vi "Madgwick Test.vi"() -> ()   [LabVIEW 2021]
uses:
  Lab 5/Lab 5 Code/Heading_TDef.ctl
  <vilib>/Platform/TimedLoop/XDataNode/timing_clust.ctl
  <vilib>/Platform/TimedLoop/XDataNode/nitl_modes.ctl
  <vilib>/Platform/TimedLoop/XDataNode/wakeup.ctl
  <vilib>/platform/TimedLoop/XDataNode/XDataNode.xnode
  <vilib>/Platform/TimedLoop/XDataNode/XDNodeRunTimeDep.lvlib
  Labview MadgwickAhrs/MadgwickOrientationFilter.lvlib
panel:
  out "Count":i32
  out "OrthogonalMatrix":dbl[][](array[numeric])
  out "Madgwick Conversion":cluster{"X":sgl, "Y":sgl, "Z":sgl}(graph)
  out "# elements in queue":i32
  out "Output Producer":dbl[][](array[numeric])
  out "Input Consumer":dbl[][](array[numeric])
  out "Quaternion":dbl[](array[numeric])
  out "Waveform Chart":waveform(dbl)[](graph)
  out "Gyro Output Offset Array (int)":i16[](array[numeric])
  in  "error in (no error)":errorcluster
  out "Mag Flux (uT)":T1(graph)
  out "Heading Output (Str)":T2
  out "Heading":dbl
  in  "Reset Gyro":bool
  out "Acceleration (g)":T3(graph)
  out "Velocity":T1(graph)
  out "Gyro Integration":T3(graph)
  out "Acceleration (ms^2)":dbl[](array[numeric])
  out "Velocity Cluster Out":cluster{i16, i16, i16}
  out "Rotation Cluster Out":T4
  out "error out":errorcluster
  in  "stop":bool
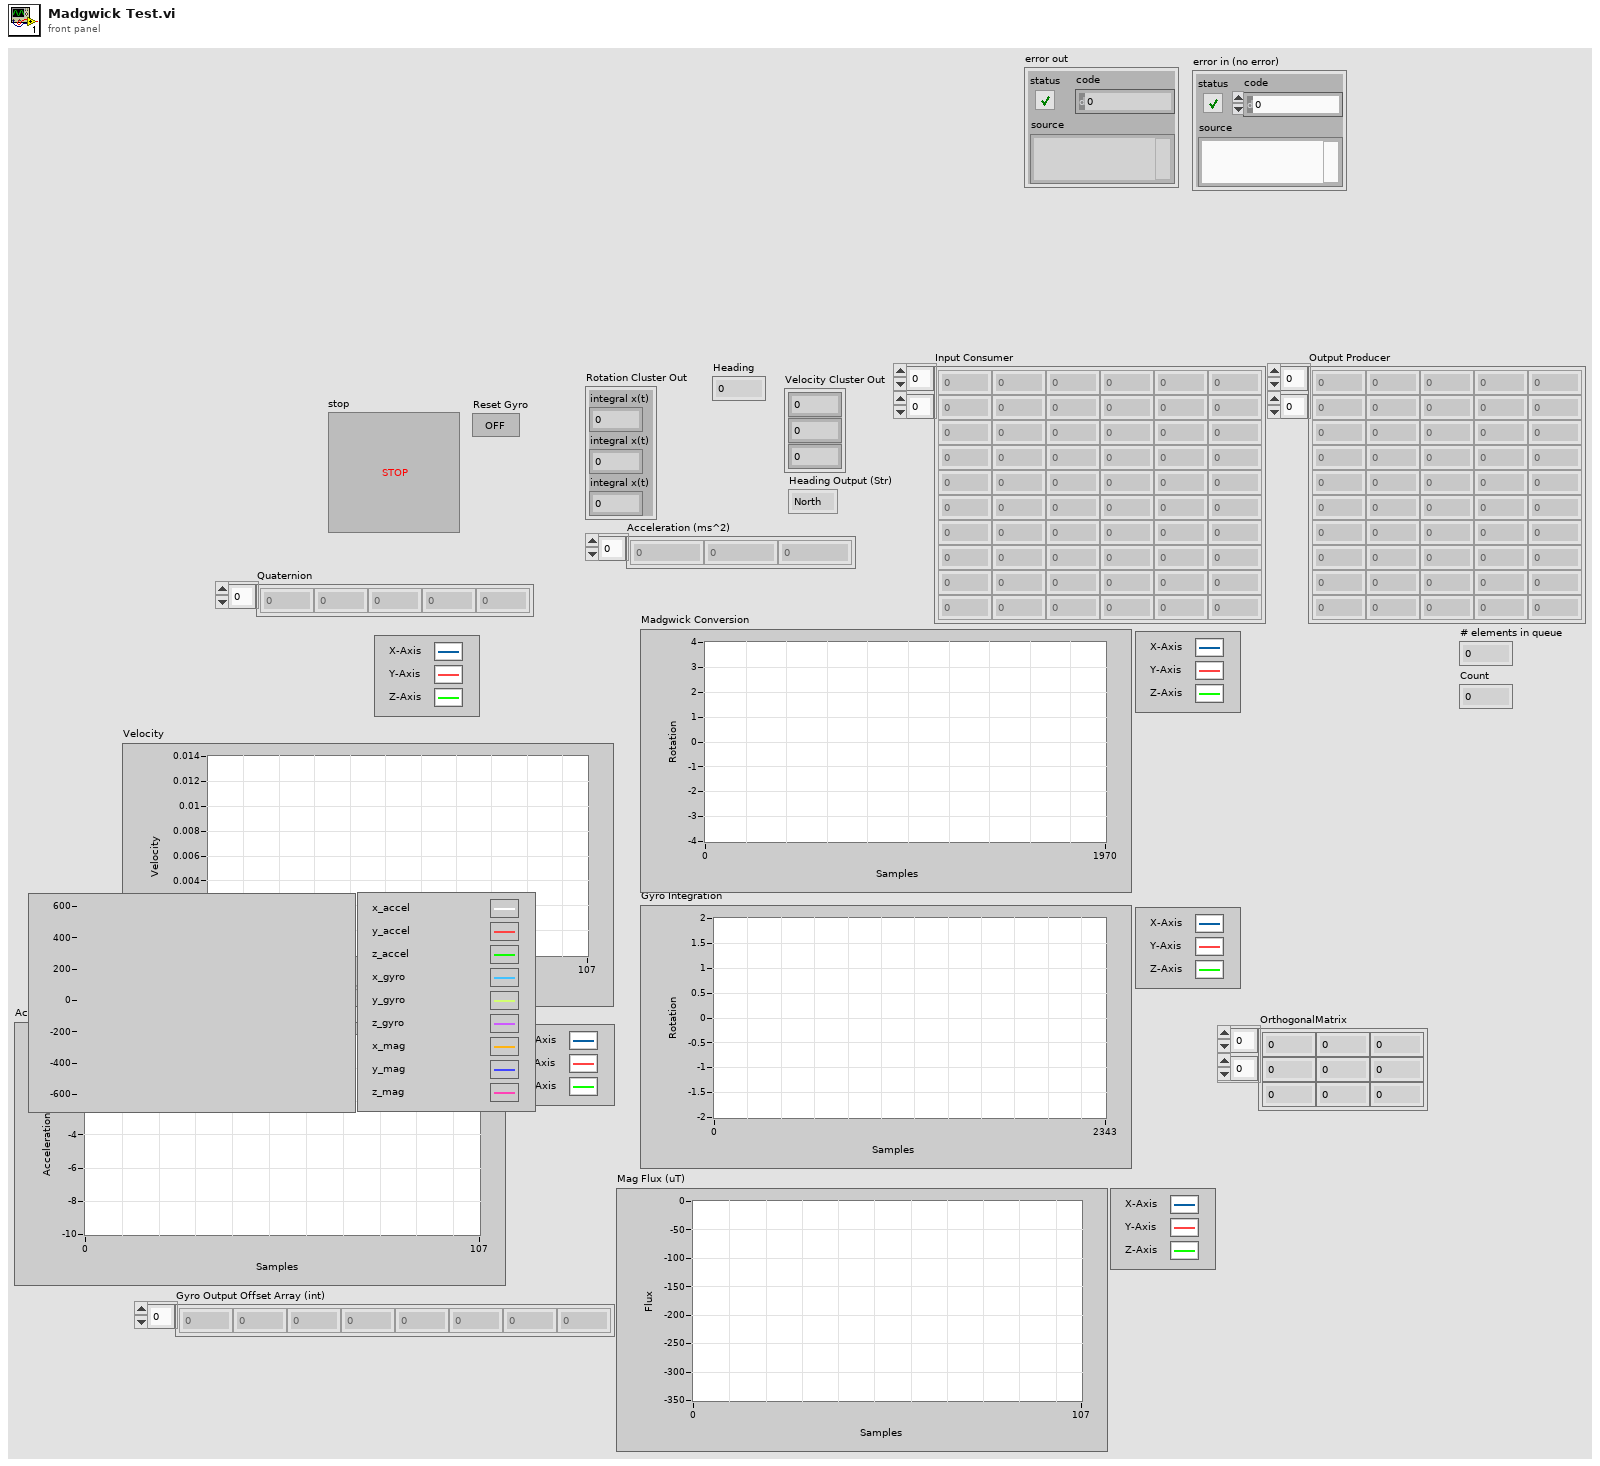
[diagram p1: front panel]
types:
  T1 = cluster{"Velocity":dbl, "Velocity":dbl, "Velocity":dbl}
  T2 = typedef "Heading_TDef.ctl" = enum16{"North ", "North East", "East", "Southeast", "South", "Southwest", "West", "Northwest"}
  T3 = cluster{"X-Axis":dbl, "Y-Axis":dbl, "Z-Axis":dbl}
  T4 = cluster{"integral x(t)":dbl, "integral x(t)":dbl, "integral x(t)":dbl}
  T5 = typedef "I2C.lvlib/I2C Reference.ctl" = cluster{"myRIO Reference":T6, "I2C Channels Enum":T10, "I2C Configuration":T11}
  T6 = typedef "myRIO Generic Hardware Reference.ctl" = cluster{"myRIO Model":T7, "myRIO Hardware Reference":T8}
  T7 = typedef "Hardware Version Enum.ctl" = enum16{"Unknown", "myRIO-1900", "myRIO-1950", "roboRIO", "NI ELVIS RIO CM", "ELVIS III"}
  T8 = typedef "myRIO v1.0 Reference.ctl" = cluster{"Generic FPGA Reference":T9, "Allow multiple opens":bool}
  T9 = typedef "Generic FPGA Reference.ctl" = refnum<k20>
  T10 = typedef "I2C Channels Enum.ctl" = enum16{"Not Connected", "A/I2C", "B/I2C", "I2C/I2C"}
  T11 = typedef "I2C.lvlib/I2C Configuration.ctl" = cluster{"I2C Transfer Rate":T12}
  T12 = typedef "I2C.lvlib/I2C Transfer Rate.ctl" = enum16{"Standard mode (100 kbps)", "Fast mode (400 kbps)"}
  T13 = typedef "XDNodeRunTimeDep.lvlib/timing_clust.ctl" = cluster{"Expected End [f-1]":u64, "Actual End [f-1]":u64, "Finished Late? [f-1]":bool, "Expected End [i-1]":u64, "Actual End [i-1]":u64, "Finished Late? [i-1]":bool, "Expected Start [i]":u64, "Actual Start [i]":u64, "Expected Start [f]":u64, "Actual Start [f]":u64, "Source Name":string, "Structure Name":string, "Period":i64, "Deadline":i64, "Offset":i64, "Start":i64, "Priority":i32, "Timeout":i32, "Mode":T14, "Wakeup Reason":T15, "Error":errorcluster, "Source Type":string, "Secondary Source Type":string, "Global End Time":u64, "Global Start Time":u64, "Frame Duration":u64, "Iteration Duration":u64, "Assigned CPU":i32, "I/O Scan Engine Mode":u32}
  T14 = typedef "XDNodeRunTimeDep.lvlib/nitl_modes.ctl" = enum32{"No Change", "Process missed periods, maintain original phase", "Discard missed periods, maintain original phase", "Process missed periods, ignore original phase", "Discard missed periods, ignore original phase"}
  T15 = typedef "XDNodeRunTimeDep.lvlib/wakeup.ctl" = enum32{"Normal", "Aborted", "Asynchronous wakeup", "Timing source error", "Timed loop error", "Timeout"}
  T16 = cluster{"X Flux (mG)":dbl, "Y Flux (mG)":dbl, "Z Flux (mG)":dbl}
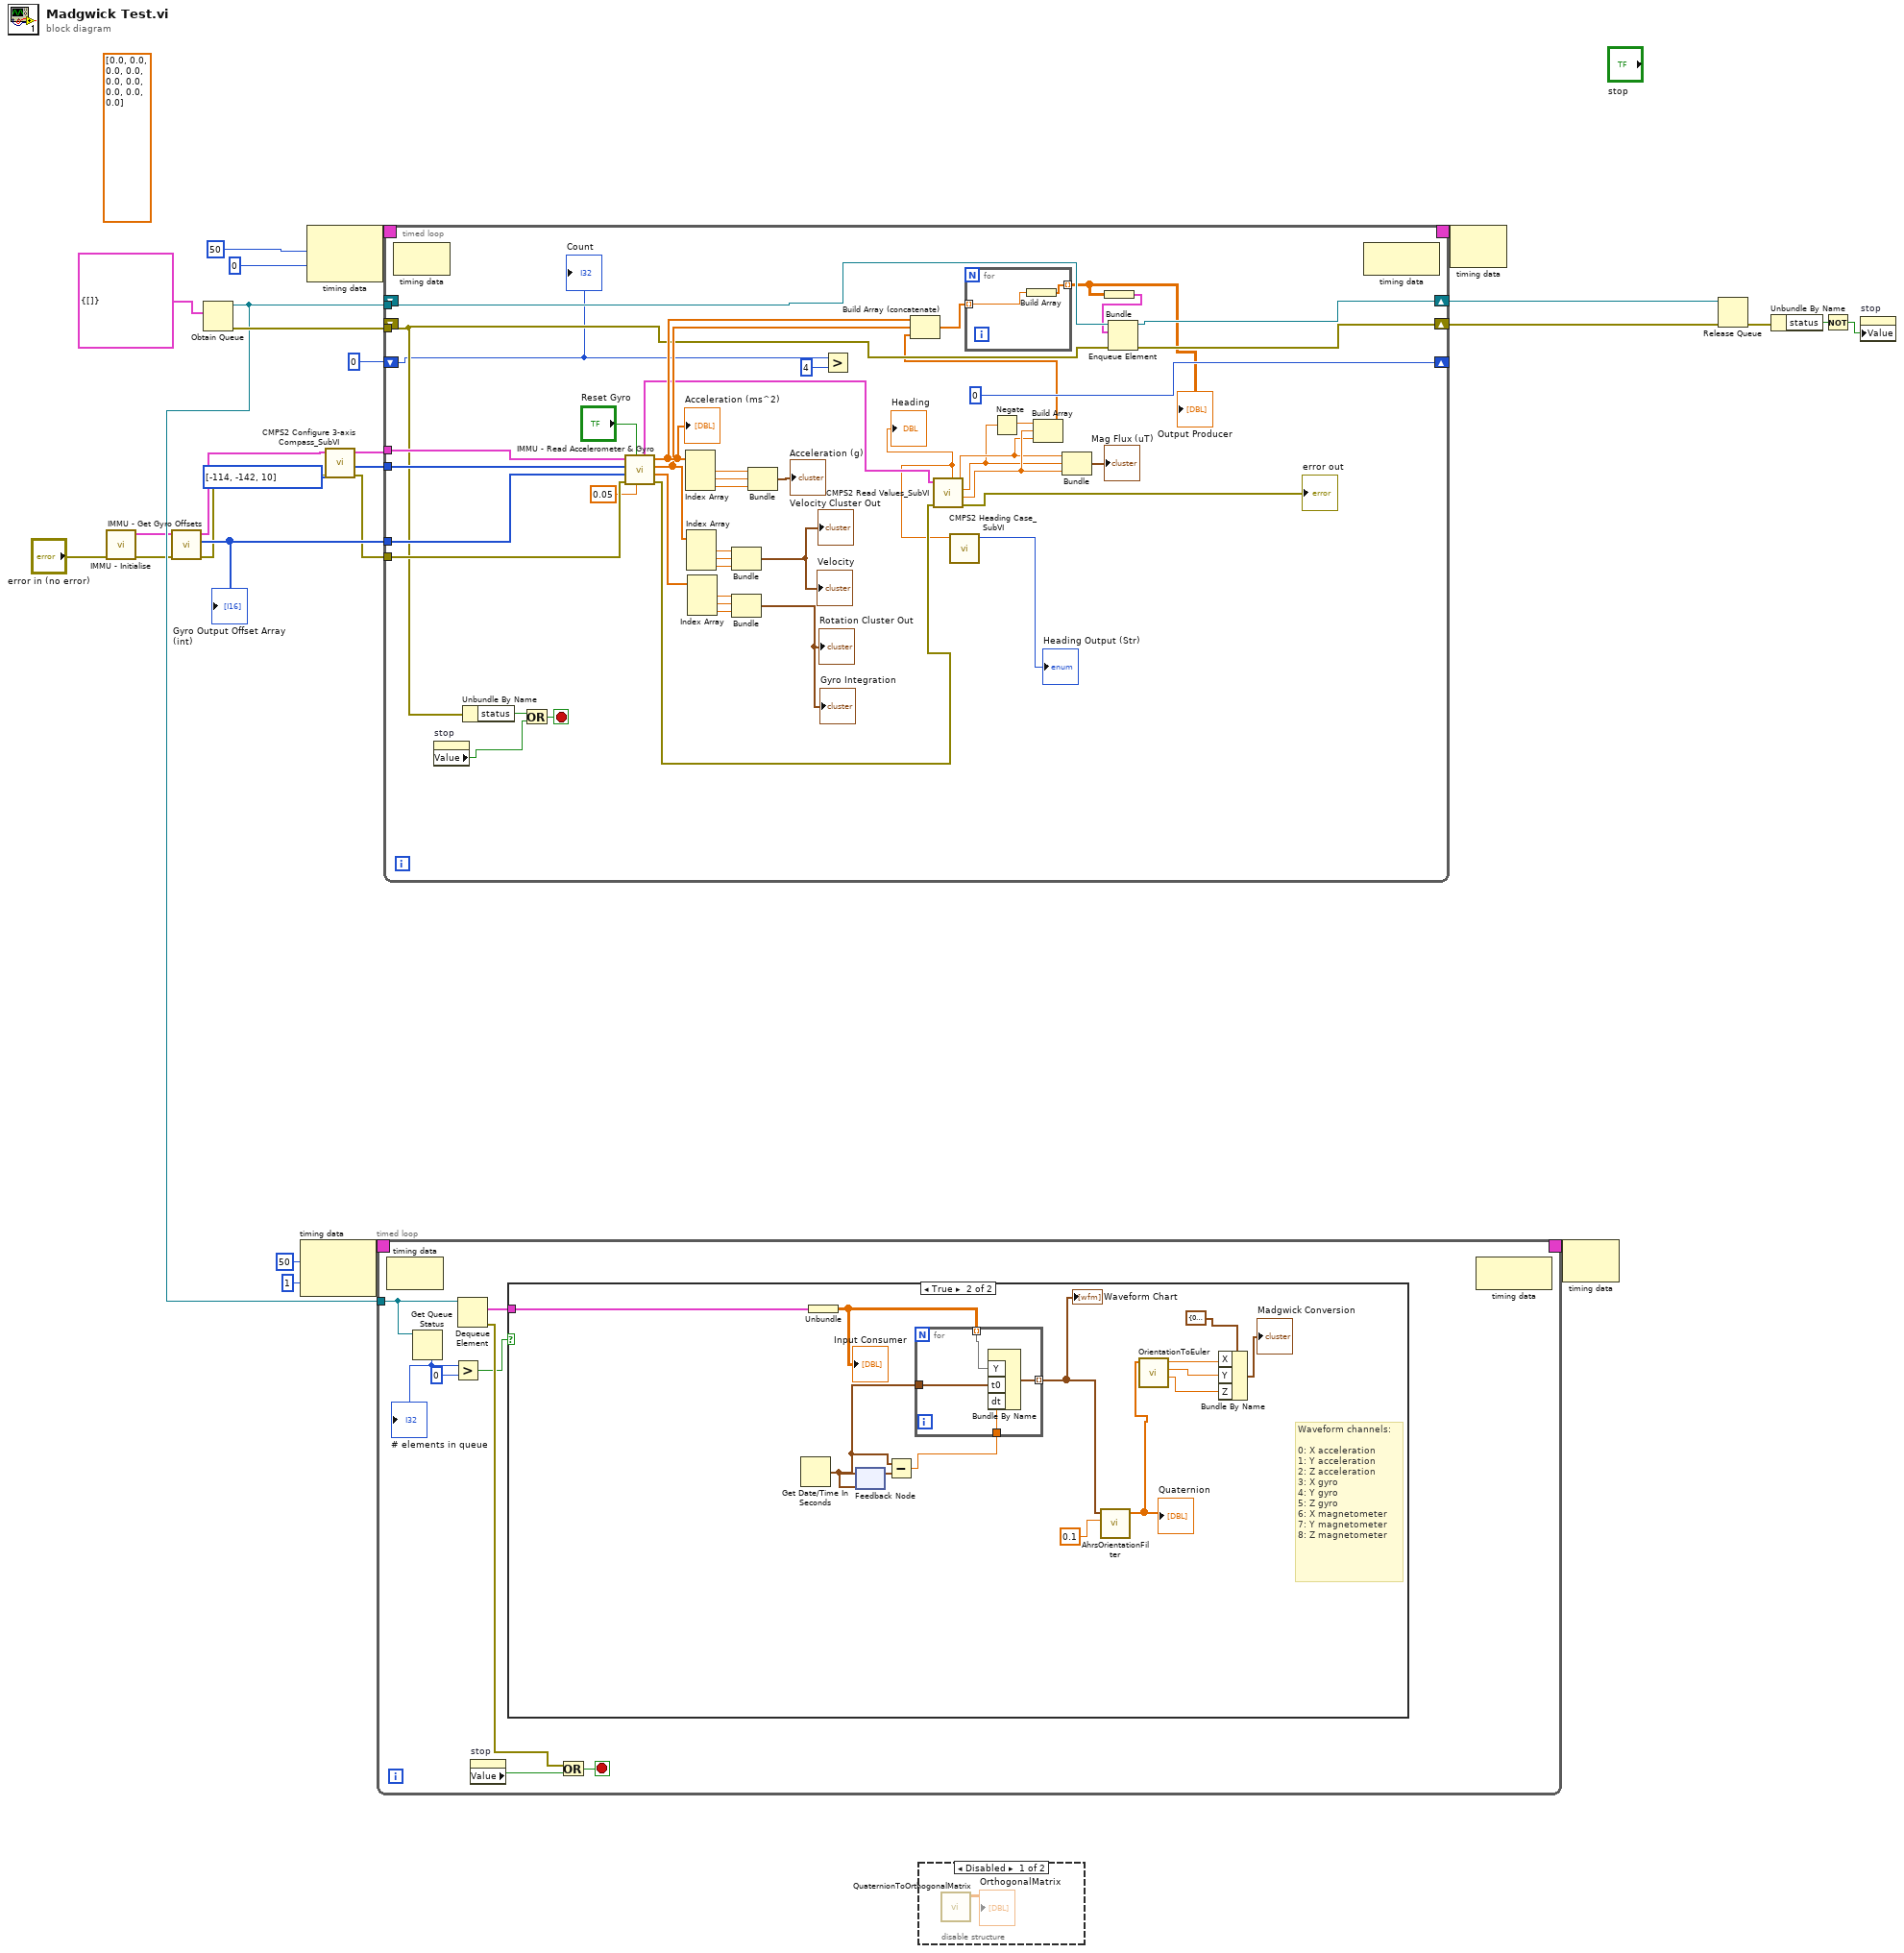
[diagram p0: block diagram]
diagram:
  (unwired) dbl[][] [[0.0], [0.0], [0.0], [0.0], [0.0], [0.0], [0.0], [0.0], [0.0]]
  n1 = call "IMMU - Initialise.vi"("error in (no error)"="error in (no error)") -> ("error out"=w13:errorcluster, "I2C Ref Out"=w12:T5)  [unwired: 9 in]
  n2 = call "IMMU - Get Gyro Offsets.vi"("error in (no error)"=w13, "I2C Ref In"=w12) -> ("error out"=w2:errorcluster, "Output Offset Array (int)"=w10:i16[], "I2C Ref Out"=w3:T5)  [unwired: 7 in]
  "Gyro Output Offset Array (int)" <- w10
  n3 = Obtain Queue(element data type=cluster{dbl[][]} {[]}) -> (queue out=w18:refnum<queue>, error out=w19:errorcluster)  [unwired: 4 in, 1 out]
  n4 = node-c288(i64 50 ("Period"), 1 ("Processor")) -> (w24:T13)
  n5 = node-c288(i64 50 ("Period"), 0 ("Processor")) -> (w26:T13)
  n6 = call "CMPS2 Configure 3-axis Compass_SubVI.vi"("error in (no error)"=w2, "I2C Ref In"=w3) -> ("error out"=w1:errorcluster, "I2C Ref Out"=w4:T5)  [unwired: 8 in]
  n7 = timed-loop {
    timing: w24 -> [_]
    timing-out: [_] -> w23
    tunnel: w18 -> [w32]
    stop <- w31 stop-if-true
    n8 = node-c288() -> ()  [unwired: 1 in, 1 out]
    n9 = Get Queue Status(queue=w32) -> (# elements in queue=w33:i32)  [unwired: 2 in, 7 out]
    "# elements in queue" <- w33
    n10 = Greater?(x=w33, y=0) -> (0:w27:bool)
    n11 = Dequeue Element(queue=w32) -> (element=w28:cluster{dbl[][]}, error out=w30:errorcluster)  [unwired: 2 in, 2 out]
    n12 = property on="stop" class="Bool (strict)"() -> ("Value"=w29:bool)  [unwired: 2 in, 2 out]
    n13 = case shown="True" w27 {
      tunnel: w28 -> [_ w42]
      frame False {
      }
      frame True {
        # "Waveform channels:\n\n0: X acceleration\n1: Y acceleration\n2: Z acceleration\n3: X gyro\n4: Y gyro\n5: Z gyro\n6: X magnetometer\n7: Y magnetometer\n8: Z magnetometer"
        n14 = Get Date/Time In Seconds() -> (seconds since 1Jan1904=w45:timestamp)
        n15 = Unbundle(w42) -> (w41:dbl[][])
        "Input Consumer" <- w41
        n16 = feedback #1(w45) -> (w44:timestamp)
        n17 = feedback-in #1(w45) -> ()
        n18 = Subtract(x=w45, y=w44) -> (x-y=w46:dbl)
        n19 = for {
          tunnel: w45 -> [w51]
          tunnel: w46 -> [w50]
          tunnel: [w49] -> w47 mode=indexing
          tunnel: w41 -> [w48] mode=indexing
          n20 = Bundle By Name("Y"=w48, "t0"=w51, "dt"=w50) -> (w49:waveform(dbl))  [unwired: 1 in]
        }
        "Waveform Chart" <- w47
        n21 = call "AhrsOrientationFilter.vi"("Beta"=0.1, "WaveformArray"=w47) -> ("Quaternion"=w40:dbl[])  [unwired: 9 in]
        "Quaternion" <- w40
        n22 = call "OrientationToEuler.vi"("Quaternion"=w40) -> ("rho"=w37:dbl, "theta"=w38:dbl, "xi"=w39:dbl)  [unwired: 8 in]
        n23 = Bundle By Name(cluster=cluster{"X":sgl, "Y":sgl, "Z":sgl} {"X"=0.0, "Y"=0.0, "Z"=0.0} ("Axis"), "X"=w39, "Y"=w38, "Z"=w37) -> (→"Madgwick Conversion":cluster{"X":sgl, "Y":sgl, "Z":sgl})
      }
    }
    n24 = Or(x=w30, y=w29) -> (x .or. y?=w31:bool)
    n25 = node-c288() -> ()  [unwired: 1 in, 1 out]
  }
  n26 = timed-loop {
    timing: w26 -> [_]
    timing-out: [_] -> w25
    tunnel: w18 -> [w73]
    tunnel: w19 -> [w72]
    shift-right: [w74] -> w17
    shift-left: _ -> [_]
    shift-right: [w67] -> w16
    shift-left: _ -> [_]
    tunnel: i16[] [-114, -142, 10] ("Accel Offset Array In") -> [w89]
    tunnel: w10 -> [w88]
    tunnel: w4 -> [w87]
    tunnel: w1 -> [w86]
    shift-right: [0] -> _
    shift-left: 0 -> [w68]
    stop <- w98 stop-if-true
    n27 = node-c288() -> ()  [unwired: 1 in, 1 out]
    n28 = property on="stop" class="Bool (strict)"() -> ("Value"=w96:bool)  [unwired: 2 in, 2 out]
    n29 = Unbundle By Name(w72) -> ("status"=w97:bool)
    n30 = Or(x=w97, y=w96) -> (x .or. y?=w98:bool)
    n31 = call "IMMU - Read Accelerometer & Gyro.vi"("dt"=0.05, "Reset Gyro"="Reset Gyro", "error in (no error)"=w86, "Gyro Offset Array In"=w88, "Accel Offset Array In"=w89, "I2C Ref In"=w87) -> ("error out"=w63:errorcluster, "Gyro Rotation Out (degrees)"=w90:dbl[], "Gyro Rotational Velocity Out (deg/s)"=w75:dbl[], "Output Acceleration Array (ms^2)"=w76:dbl[], "I2C Ref Out"=w62:T5)  [unwired: 1 in]
    "Acceleration (ms^2)" <- w76
    n32 = Index Array(array=w76) -> (element #1=w82:dbl, element #2=w81:dbl, element #3=w80:dbl)  [unwired: 3 in]
    n33 = Index Array(array=w75) -> (element #1=w79:dbl, element #2=w78:dbl, element #3=w77:dbl)  [unwired: 3 in]
    n34 = Index Array(array=w90) -> (element #1=w95:dbl, element #2=w94:dbl, element #3=w93:dbl)  [unwired: 3 in]
    n35 = Bundle(w79, w78, w77) -> (→"Velocity Cluster Out" →"Velocity":cluster{dbl, dbl, dbl})  [unwired: 1 in]
    n36 = Bundle("integral x(t)"=w95, "integral x(t)"=w94, "integral x(t)"=w93) -> (→"Rotation Cluster Out" →"Gyro Integration":T4)  [unwired: 1 in]
    n37 = Bundle(w82, w81, w80) -> (→"Acceleration (g)":cluster{dbl, dbl, dbl})  [unwired: 1 in]
    n38 = Greater?(x=w68, y=4) -> ()  [unwired: 1 out]
    n39 = call "CMPS2 Read Values_SubVI.vi"("error in (no error)"=w63, "I2C Ref In"=w62) -> ("error out"=→"error out":errorcluster, "Z Flux (mG)"=w57:dbl, "Y Flux (mG)"=w55:dbl, "X Flux (mG)"=w56:dbl, "Heading"=w60:dbl)  [unwired: 4 in, 1 out]
    "Heading" <- w60
    n40 = call "CMPS2 Heading Case_SubVI.vi"("Numeric"=w60) -> ("Heading String 2"=→"Heading Output (Str)":T2)  [unwired: 10 in]
    n41 = Negate(x=w55) -> (-x=w54:dbl)
    n42 = Build Array(w54, w57, w56) -> (w58:dbl[])
    n43 = Build Array (concatenate)(w76, w75, w58) -> (w66:dbl[])
    n44 = for {
      tunnel: w66 -> [w99] mode=indexing
      tunnel: [w100] -> w64 mode=indexing
      n45 = Build Array(w99) -> (w100:dbl[])
    }
    "Output Producer" <- w64
    n46 = Bundle("X Flux (mG)"=w56, "Y Flux (mG)"=w55, "Z Flux (mG)"=w57) -> (→"Mag Flux (uT)":T16)  [unwired: 1 in]
    n47 = Bundle(w64) -> (w65:cluster{dbl[][]})  [unwired: 1 in]
    n48 = Enqueue Element(queue=w73, element=w65, error in (no error)=w72) -> (queue out=w67:refnum<queue>, error out=w74:errorcluster)  [unwired: 1 in, 1 out]
    n49 = node-c288() -> ()  [unwired: 1 in, 1 out]
    "Count" <- w68
  }
  n50 = disable-structure shown="Disabled" {
    frame Disabled {
      n51 = call "QuaternionToOrthogonalMatrix.vi"() -> ("OrthogonalMatrix"=→"OrthogonalMatrix":dbl[][])  [unwired: 11 in]
    }
    frame Enabled {
    }
  }
  n52 = node-c288(w25) -> ()  [unwired: 1 out]
  n53 = node-c288(w23) -> ()  [unwired: 1 out]
  n54 = Release Queue(queue=w16, error in (no error)=w17) -> (error out=w8:errorcluster)  [unwired: 1 in, 2 out]
  n55 = Unbundle By Name(w8) -> ("status"=w7:bool)
  n56 = Not(x=w7) -> (.not. x?=w6:bool)
  n57 = property on="stop" class="Bool (strict)"("Value"=w6) -> ()  [unwired: 2 in, 2 out]
